vi "Configure Peak Detection Parameters.vi"(7 "Micropulse # In":i32, 8 "error in (no error)":errorcluster, 9 "Peak Settings":T1={"Upper Threshold"=0, "Hysteresis"=enum."None", "# Peaks In Gate"=10}, 11 "Test Number":u32) -> (0 "error out":errorcluster, 3 "Test Number Out":u32, 5 "Micropulse # Out":i32)   [LabVIEW 2026, in "MicroPulse_Driver.lvlib"]
uses:
  MicroPulse_Driver.lvlib
  Data/Datatypes/MP - peak settings.ctl
  Data/Datatypes/MP - hysteresis level.ctl
  <instrlib>/Micropulse/Micropulse.lvlib
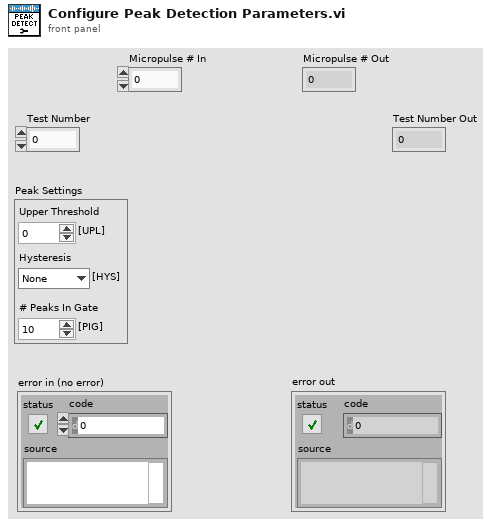
[diagram p1: front panel]
types:
  T1 = typedef "Micropulse.lvlib/MP - peak settings.ctl" = cluster{"Upper Threshold":u16, "Hysteresis":T2, "# Peaks In Gate":u16}
  T2 = typedef "Micropulse.lvlib/MP - hysteresis level.ctl" = enum16{"None", "3dB", "6dB", "9dB", "12dB"}
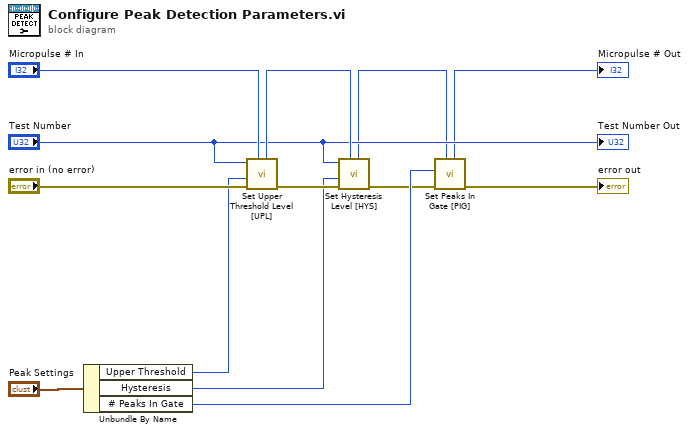
[diagram p0: block diagram]
diagram:
  n1 = Unbundle By Name("Peak Settings") -> ("Upper Threshold"=w5:u16, "Hysteresis"=w8:T2, "# Peaks In Gate"=w7:u16)
  n2 = call "Set Upper Threshold Level [UPL].vi"("Micropulse # In"="Micropulse # In", "error in (no error)"="error in (no error)", "Threshold"=w5, "Test Number"="Test Number") -> ("error out"=w12:errorcluster, "Micropulse # Out"=w9:i32)  [unwired: 6 in]
  n3 = call "Set Hysteresis Level [HYS].vi"("Micropulse # In"=w9, "error in (no error)"=w12, "Hysteresis Level"=w8, "Test Number"="Test Number") -> ("error out"=w4:errorcluster, "Micropulse # Out"=w3:i32)  [unwired: 6 in]
  n4 = call "Set Peaks In Gate [PIG].vi"("Micropulse # In"=w3, "error in (no error)"=w4, "# Peaks to report"=w7) -> ("error out"=→"error out":errorcluster, "Micropulse # Out"=→"Micropulse # Out":i32)  [unwired: 7 in]
  "Test Number Out" <- "Test Number"
